vi "1931C Commands.vi"(0 "Instrument Resource Name":refnum<visa-resource-name>, 7 "Command":u16(ring) items=["Attenuator OFF", "Attenuator ON", "Attenuator Query", "Beep OFF", "Beep ON", "Beep Query", "Clear Status Reg", "Data Query (nW)", "Echo OFF", "Echo ON", "Echo Query", "No Filter", "Analog Filter", "Digital FIlter", "Filter Query", "Hold", "Go", "Go Query", "Backlight OFF", "Backlight Medium", "Backlight High", "Backlight Query", "Set Dsplay Screen 0", "Set Display Screen 1", "Display Screen Query", "Mode DC Continuous", "Mode DC Single", "Mode Integrate", "Identification", "Auto Range", "Auto Range Query", "Signal Range 0", "Signal Range 1", "Signal Range 2", "Signal Range 3", "Signal Range 4", "Signal Range 5", "Signal Range 6", "Signal Range Query", "Store Reference", "Units W", "Units W/cm2", "Units dBm", "Units Joules", "Units Query", "Set Wavelength", "Wavelength Querry", "Mode Pesk-to-Peak Cont.", "Mode Peak-to-Peak Sing.", "Mode Query"], 9 "Wavelength":string, 11 "error in (no error)":errorcluster) -> (4 "VISA resource name out":refnum<visa-resource-name>, 6 "Bytes Read":dbl, 8 "LM Response":dbl format="%#_4g", 10 "Read String":string, 15 "error out":errorcluster {"code" format="%.0x"})   [LabVIEW 2010]
uses:
  <vilib>/Instr/_visa.llb/VISA Configure Serial Port (Instr).vi
panel:
  out "Bytes Written":dbl
  out "Write String":string
  out "Actual Numeric Resp":dbl
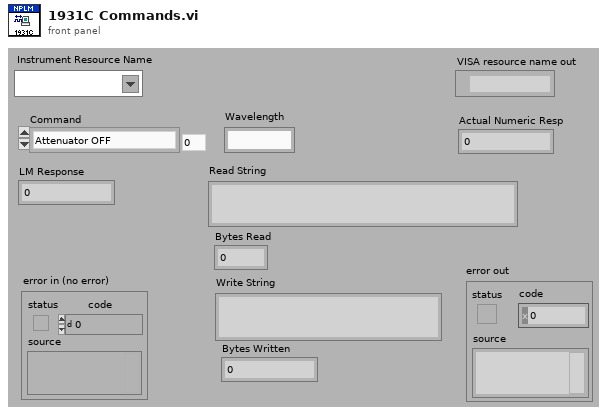
[diagram p1: front panel]
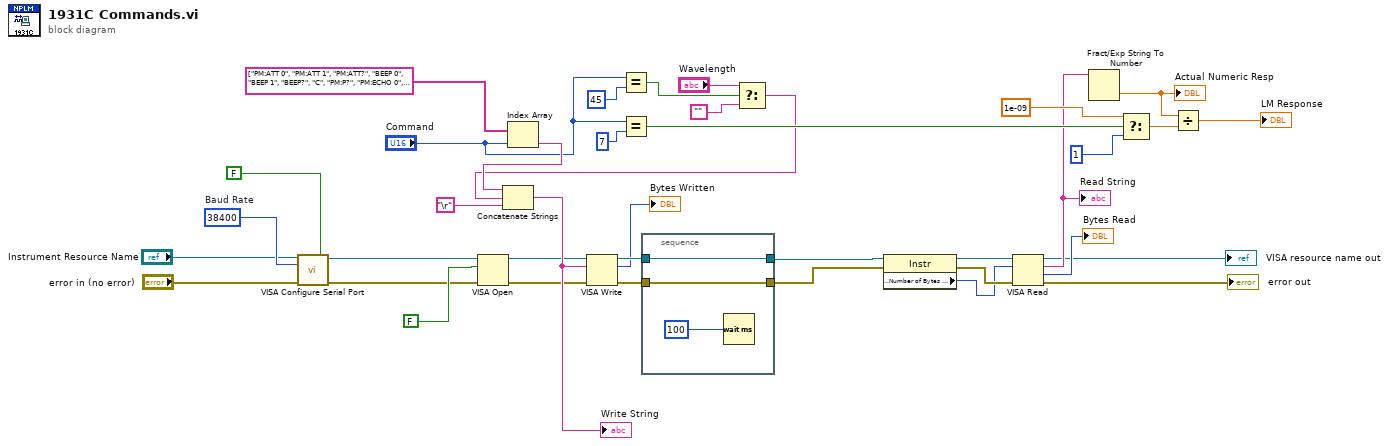
[diagram p0: block diagram]
diagram:
  w17 = 38400  # Baud Rate
  n1 = call-poly "VISA Configure Serial Port"("VISA resource name"="Instrument Resource Name", "Enable Termination\nChar (T)"=FALSE, "baud rate (9600)"=w17, "error in (no error)"="error in (no error)") -> ("VISA resource name out"=w3:refnum<visa-resource-name>, "error out"=w1:errorcluster)  [unwired: 10 in]
  n2 = VISA Open(duplicate session (F)=FALSE, error in (no error)=w1, VISA resource name=w3) -> (VISA resource name=w12:refnum<visa-resource-name>, error out=w11:errorcluster)  [unwired: 2 in]
  n3 = Index Array(array=string[] ["PM:ATT 0", "PM:ATT 1", "PM:ATT?", "BEEP 0", "BEEP 1", "BEEP?", "C", "PM:P?", "PM:ECHO 0", "PM:ECHO 1", "PM:ECHO?", "PM:FILT 0\nF1", "PM:FILT 1", "PM:FILT 2", "PM:FILT?", "PM:RUN 0", "PM:RUN 1", "PM:RUN?", "DISP:BRIGHT 0", "DISP:BRIGHT 4", "DISP:BRIGHT 7", "DISP:BRIGHT?", "DISP:SCR 0", "DISP:SCR 1", "DISP:SCR?", "PM:MODE 0", "PM:MODE 1", "PM:MODE 2", "*IDN?", "PM:AUTO 1", "PM:AUTO?", "PM:RAN 0", "PM:RAN 1", "PM:RAN 2", "PM:RAN 3", "PM:RAN 4", "PM:RAN 5", "PM:RAN 6", "PM:RAN?", "PM:REF:STO", "PM:UNIT 2", "PM:UNIT 3", "PM:UNIT 6", "PM:UNIT 4", "PM:UNIT?", "PM:L ", "PM:L?", "PM:MODE 3", "PM:MODE 4", "PM:MODE?"], index="Command") -> (element=w30:string)
  n4 = Equal?(x="Command", y=45) -> (x = y?=w19:bool)
  n5 = Equal?(x="Command", y=7) -> (x = y?=w25:bool)
  n6 = Select(t="Wavelength", s=w19, f="") -> (s? t:f=w18:string)
  n7 = Concatenate Strings(w30, w18, "\r") -> (w13:string)
  "Write String" <- w13
  n8 = VISA Write(VISA resource name=w12, write buffer=w13, error in (no error)=w11) -> (VISA resource name out=w34:refnum<visa-resource-name>, return count=→"Bytes Written":u32, error out=w33:errorcluster)
  n9 = stacked-sequence {
    tunnel: w34 -> [w41]
    tunnel: [w41] -> w10
    tunnel: [w40] -> w9
    tunnel: w33 -> [w40]
    frame #0 {
      n10 = Wait (ms)(milliseconds to wait=u32 100 ("delay before read (ms)")) -> ()  [unwired: 1 out]
    }
  }
  n11 = property class="Instr"(reference=w10, error in=w9) -> (reference out=w38:refnum<visa-resource-name>, error out=w37:errorcluster, "Serial Settings:Number of Bytes at Serial Port"=w35:u32)
  n12 = VISA Read(VISA resource name=w38, byte count=w35, error in (no error)=w37) -> (VISA resource name out=→"VISA resource name out":refnum<visa-resource-name>, read buffer=w15:string, return count=→"Bytes Read":u32, error out=→"error out":errorcluster)
  "Read String" <- w15
  n13 = Fract/Exp String To Number(string=w15) -> (number=w32:dbl)  [unwired: 3 in, 1 out]
  "Actual Numeric Resp" <- w32
  n14 = Select(t=1e-09, s=w25, f=1) -> (s? t:f=w29:dbl)
  n15 = Divide(x=w32, y=w29) -> (x/y=→"LM Response":dbl)
